vi "QNET_ROTPEN_Swing_Up_Control.vi"(0 "theta_dot (rad/s)":dbl, 1 "alpha_dot (rad/s)":dbl, 2 "alpha_full (rad)":dbl, 3 "Swing-Up Control Parameters":T2={"mu (m/s^2/J)"=375.0, "Er (mJ)"=20.0, "max accel (m/s^2)"=35.0, "enable"=FALSE} caption="Control Parameters" {"Er (mJ)" min=0.0 max=500.0 step=5.0 format="%_3f"; "mu (m/s^2/J)" min=0.0 max=750.0 step=5.0 format="%_3f"}, 4 "Model Parameters":T1={"Mp"=0.027000000700354576, "lp"=0.15299999713897705, "r"=0.08259999752044678, "Jp"=0.0005089999758638442, "Jeq"=0.0001230000052601099, "Kt"=0.02800000086426735, "Rm"=3.299999952316284, "Bp"=0.0, "Beq"=0.0, "Marm"=0.02800000086426735} {"Marm" min=0.0 step=0.0010000000474974513 format="%_3f"; "Beq" min=0 max=0.01 format="%_3g"; "Bp" min=0 max=0.01 format="%_3g"; "Rm" min=0.0 max=5.0 step=0.05000000074505806 format="%_3f"; "Kt" min=0.0 max=0.10000000149011612 step=0.0010000000474974513 format="%_3f"; "Jeq" min=0.0 max=0.0010000000474974513 step=9.999999747378752e-06 format="%_3g"; "Jp" min=0.0 max=0.0010000000474974513 step=9.999999747378752e-06 format="%_3g"; "r" min=0.0 max=0.20000000298023224 step=0.0010000000474974513 format="%_3f"; "lp" min=0.0 max=1.0 step=0.0010000000474974513 format="%#_3f"; "Mp" min=0.0 step=0.0010000000474974513 format="%_3f"}) -> (5 "Vm (V)":dbl, 6 "E (mJ)":dbl)   [LabVIEW 2010]
panel:
  # "kg"
  # "m"
  # "kg"
  # "m"
  # "kg.m^2"
  # "kg.m^2"
  # "N.m/A"
  # "ohm"
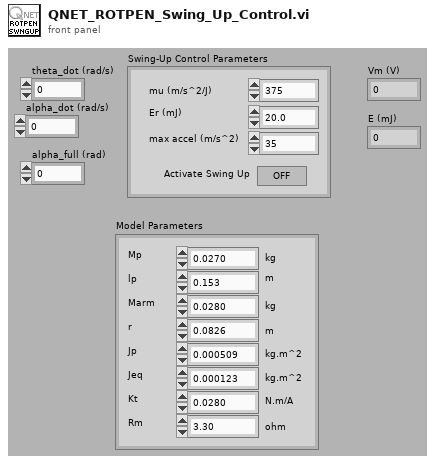
[diagram p1: front panel]
types:
  T1 = cluster{"Mp":dbl, "lp":dbl, "r":dbl, "Jp":dbl, "Jeq":dbl, "Kt":dbl, "Rm":dbl, "Bp":sgl, "Beq":sgl, "Marm":dbl}
  T2 = cluster{"mu (m/s^2/J)":dbl, "Er (mJ)":dbl, "max accel (m/s^2)":dbl, "enable":bool}
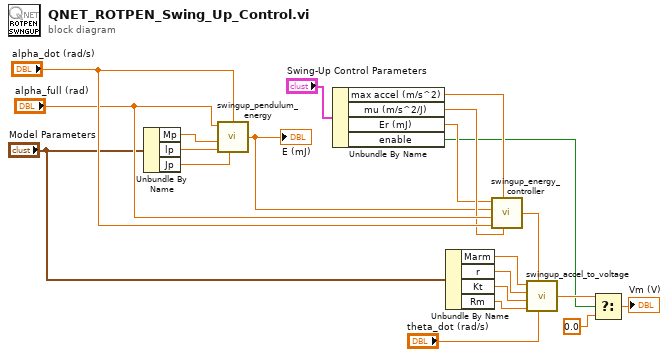
[diagram p0: block diagram]
diagram:
  n1 = Unbundle By Name("Model Parameters") -> ("Mp"=w13:dbl, "lp"=w14:dbl, "Jp"=w12:dbl)
  n2 = call "swingup_pendulum_energy.vi"("alpha_full (rad)"="alpha_full (rad)", "alpha_dot (rad/s)"="alpha_dot (rad/s)", "mp (kg)"=w13, "lp (m)"=w14, "Jp (kg.m^2)"=w12) -> ("E (mJ)"=w18:dbl)
  "E (mJ)" <- w18
  n3 = Unbundle By Name("Swing-Up Control Parameters") -> ("max accel (m/s^2)"=w16:dbl, "mu (m/s^2/J)"=w19:dbl, "Er (mJ)"=w17:dbl, "enable"=w4:bool)
  n4 = Unbundle By Name("Model Parameters") -> ("Marm"=w7:dbl, "r"=w8:dbl, "Kt"=w9:dbl, "Rm"=w10:dbl)
  n5 = call "swingup_energy_controller.vi"("mu (m/s^2/J)"=w19, "max_u (m/s^2)"=w16, "alpha_dot (rad/s)"="alpha_dot (rad/s)", "alpha_full (rad)"="alpha_full (rad)", "E (mJ)"=w18, "Er (mJ)"=w17) -> ("u (m/s^2)"=w15:dbl)
  n6 = call "swingup_accel_to_voltage.vi"("theta_dot (rad/s)"="theta_dot (rad/s)", "u (m/s^2)"=w15, "Rm (ohms)"=w10, "Kt (N.m/A)"=w9, "r (m)"=w8, "m_arm (kg)"=w7) -> ("Vm (V)"=w6:dbl)
  n7 = Select(t=w6, s=w4, f=0.0) -> (s? t:f=→"Vm (V)":dbl)
